vi "OutputLimeLight.vi"   [LabVIEW 2020]
doc: "This VI sends commands to the LimeLight camera."
uses:
  bed327a2-98d3-4965-916e-7305edcf582b.vi
  9959ab12-4f3e-4c63-8bb4-e3e2fa624083.vi
  bed327a2-98d3-4965-916e-7305edcf582b.vi/77c742ae-e671-49bb-a825-a6e8cebc9f63.vi
  9959ab12-4f3e-4c63-8bb4-e3e2fa624083.vi/77c742ae-e671-49bb-a825-a6e8cebc9f63.vi
  <vilib>/Rock Robotics/Network Tables/NT Read Number.vi
  outputs.vi
  driverdata.vi
  <vilib>/Rock Robotics/Network Tables/NT Write Value.vi
  <vilib>/Rock Robotics/Network Tables/NT Write Number.vi
types:
  T1 = enum16{"Boot Up", "Camera Override", "HUB Targeting", "CARGO Tracking"}
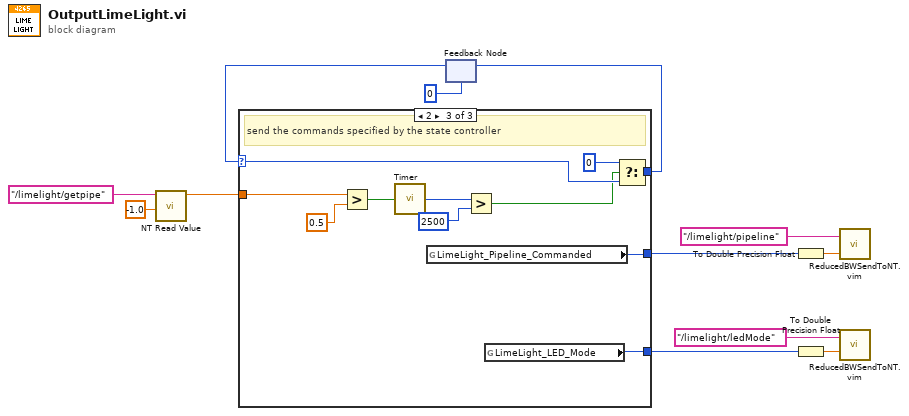
[diagram p0: block diagram]
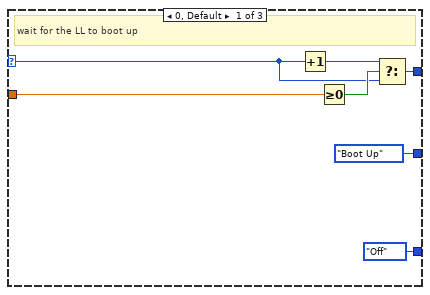
[diagram p2: hidden frame]
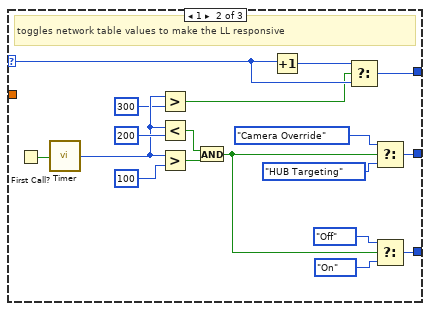
[diagram p3: hidden frame]
diagram:
  n1 = call-poly <vilib>:"NT Read Value.vi"("Default Value"=-1.0, "Name"="/limelight/getpipe") -> ("Numeric"=w1:dbl)  [unwired: 8 in, 1 out]
  n2 = feedback #1(0) -> (w9:i32)
  n3 = case shown="2" w9 {
    selector: w9 -> [w17 w36 w46]
    tunnel: [w16 w35 w47] -> w10
    tunnel: [T1."Boot Up" w20 w38] -> w5
    tunnel: [enum16{"Pipeline Setting", "Off", "Blink", "On"}."Off" ("LimeLight_LED_Mode") w21 w48] -> w4
    tunnel: w1 -> [w13 _ w44]
    frame 0, Default {
      # "wait for the LL to boot up"
      n4 = Increment(x=w17) -> (x+1=w18:i32)
      n5 = Greater Or Equal To 0?(x=w13) -> (x >= 0?=w19:bool)
      n6 = Select(t=w18, s=w19, f=w17) -> (s? t:f=w16:i32)
    }
    frame 1 {
      # "toggles network table values to make the LL responsive"
      n7 = First Call?() -> (First Call?: T/F=w34:bool)
      n8 = call "Timer.vi"("Reset Timer"=w34) -> ("Time (ms)"=w27:u32)
      n9 = Greater?(x=w27, y=u32 300) -> (0:w25:bool)
      n10 = Less?(x=w27, y=u32 200) -> (x < y?=w30:bool)
      n11 = Greater?(x=w27, y=u32 100) -> (0:w32:bool)
      n12 = And(x=w30, y=w32) -> (x .and. y?=w24:bool)
      n13 = Increment(x=w36) -> (x+1=w37:i32)
      n14 = Select(t=w37, s=w25, f=w36) -> (s? t:f=w35:i32)
      n15 = Select(t=T1."Camera Override", s=w24, f=T1."HUB Targeting") -> (s? t:f=w20:T1)
      n16 = Select(t=enum16{"Pipeline Setting", "Off", "Blink", "On"}."Off" ("LimeLight_LED_Mode"), s=w24, f=enum16{"Pipeline Setting", "Off", "Blink", "On"}."On" ("LimeLight_LED_Mode")) -> (s? t:f=w21:enum16{"Pipeline Setting", "Off", "Blink", "On"})
    }
    frame 2 {
      # "send the commands specified by the state controller"
      n17 = Greater?(x=w44, y=0.5 ("Numeric")) -> (0:w42:bool)
      n18 = call "Timer.vi"("Reset Timer"=w42) -> ("Time (ms)"=w41:u32)
      n19 = global read "outputs.vi" "LimeLight_Pipeline_Commanded"() -> (w38:T1)
      n20 = Greater?(x=w41, y=u32 2500) -> (0:w39:bool)
      n21 = global read "outputs.vi" "LimeLight_LED_Mode"() -> (w48:enum16{"Pipeline Setting", "Off", "Blink", "On"})
      n22 = Select(t=0, s=w39, f=w46) -> (s? t:f=w47:i32)
    }
  }
  n23 = feedback-in #1(w10) -> ()
  n24 = To Double Precision Float(number=w5) -> (double precision float=w7:dbl)
  n25 = To Double Precision Float(number=w4) -> (double precision float=w12:dbl)
  n26 = call "ReducedBWSendToNT.vim"("Value In"=w7, "NT Name"="/limelight/pipeline" ("Name")) -> ()  [unwired: 1 out]
  n27 = call "ReducedBWSendToNT.vim"("Value In"=w12, "NT Name"="/limelight/ledMode" ("Name")) -> ()  [unwired: 1 out]
